vi "X,Y,Z轴坐标查询.vi"(1 "细分设置":dbl, 2 "查询坐标轴":string, 3 "串口通信端口":refnum<visa-resource-name>) -> (0 "坐标(mm)":dbl)   [LabVIEW 2016]
panel:
  # "XYZ轴坐标查询"
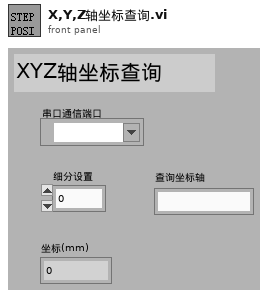
[diagram p1: front panel]
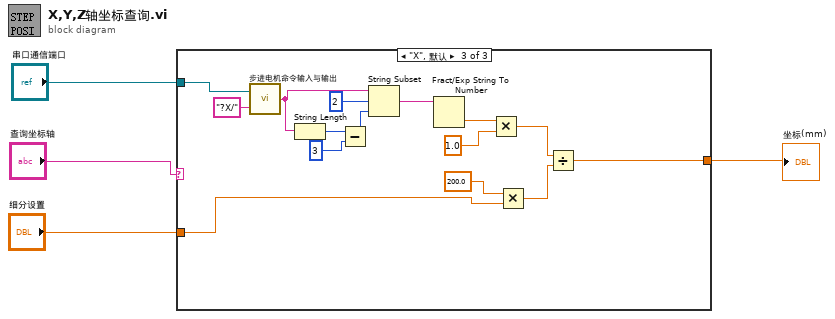
[diagram p0: block diagram]
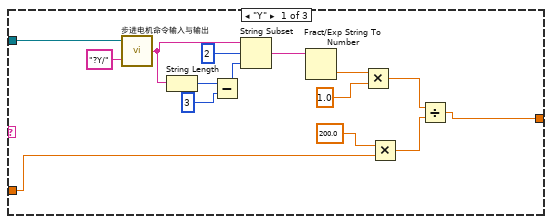
[diagram p2: hidden frame]
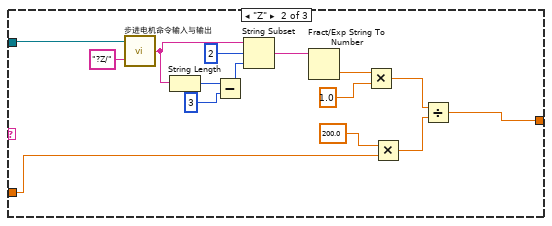
[diagram p3: hidden frame]
diagram:
  n1 = case shown="\"X\", 默认" "查询坐标轴" {
    tunnel: "串口通信端口" -> [w7 w23 w37]
    tunnel: "细分设置" -> [w6 w22 w36]
    tunnel: [w5 w20 w35] -> w1
    frame "Y" {
      n2 = call "步进电机命令输入与输出.vi"("输入字符串"="?Y/", "串口通信端口"=w7) -> ("返回字符串"=w12:string)
      n3 = String Length(string=w12) -> (length=w10:i32)
      n4 = Subtract(x=w10, y=3) -> (x-y=w13:i32)
      n5 = String Subset(string=w12, offset (0)=2 ("偏移量(0)"), length (rest)=w13) -> (substring=w14:string)
      n6 = Fract/Exp String To Number(string=w14) -> (number=w15:dbl)  [unwired: 4 out]
      n7 = Multiply(x=w15, y=1.0) -> (x*y=w19:dbl)
      n8 = Multiply(x=200.0, y=w6) -> (x*y=w18:dbl)
      n9 = Divide(x=w19, y=w18) -> (x/y=w5:dbl)
    }
    frame "Z" {
      n10 = call "步进电机命令输入与输出.vi"("输入字符串"="?Z/", "串口通信端口"=w23) -> ("返回字符串"=w28:string)
      n11 = String Length(string=w28) -> (length=w26:i32)
      n12 = Subtract(x=w26, y=3) -> (x-y=w29:i32)
      n13 = String Subset(string=w28, offset (0)=2 ("偏移量(0)"), length (rest)=w29) -> (substring=w30:string)
      n14 = Fract/Exp String To Number(string=w30) -> (number=w31:dbl)  [unwired: 4 out]
      n15 = Multiply(x=w31, y=1.0) -> (x*y=w34:dbl)
      n16 = Multiply(x=200.0, y=w22) -> (x*y=w21:dbl)
      n17 = Divide(x=w34, y=w21) -> (x/y=w20:dbl)
    }
    frame "X", Default {
      n18 = call "步进电机命令输入与输出.vi"("输入字符串"="?X/", "串口通信端口"=w37) -> ("返回字符串"=w45:string)
      n19 = String Length(string=w45) -> (length=w47:i32)
      n20 = Subtract(x=w47, y=3) -> (x-y=w44:i32)
      n21 = String Subset(string=w45, offset (0)=2 ("偏移量(0)"), length (rest)=w44) -> (substring=w43:string)
      n22 = Fract/Exp String To Number(string=w43) -> (number=w42:dbl)  [unwired: 4 out]
      n23 = Multiply(x=w42, y=1.0) -> (x*y=w38:dbl)
      n24 = Multiply(x=200.0, y=w36) -> (x*y=w39:dbl)
      n25 = Divide(x=w38, y=w39) -> (x/y=w35:dbl)
    }
  }
  "坐标(mm)" <- w1
